vi "Status.vi"(8 "error in (no error)":errorcluster, 11 "Agitator Module State Cluster":T1={"State"=enum."Idle", "Start Time"=timestamp(0 s since 1904-01-01), "Current Time"=timestamp(0 s since 1904-01-01), "Agitator Module Config"={"GUID"="", "Drop Coords"={"Horizontal"=0, "Vertical"=0}, "Process Name"="", "User name"="", "Queue Name"="", "Settings"={"Cycle Period"=500.0, "Agitator Type"="", "Setpoint (µm)"=0.0, "IKA EUROSTAR Settings"={"VISA resource name"="", "Simulated?"=FALSE}}, "Load Count"=0}, "Output Error"=FALSE, "Log Started"=FALSE, "First Iteration"=FALSE, "Data"={"Agitator rpm Value"=0.0}, "Agitator On?"=enum."Off"}) -> (0 "error out":errorcluster, 3 "Agitator Module State Cluster":T1={"State"=enum."Idle", "Start Time"=timestamp(0 s since 1904-01-01), "Current Time"=timestamp(0 s since 1904-01-01), "Agitator Module Config"={"GUID"="", "Drop Coords"={"Horizontal"=0, "Vertical"=0}, "Process Name"="", "User name"="", "Queue Name"="", "Settings"={"Cycle Period"=500.0, "Agitator Type"="", "Setpoint (µm)"=0.0, "IKA EUROSTAR Settings"={"VISA resource name"="", "Simulated?"=FALSE}}, "Load Count"=0}, "Output Error"=FALSE, "Log Started"=FALSE, "First Iteration"=FALSE, "Data"={"Agitator rpm Value"=0.0}, "Agitator On?"=enum."Off"})   [LabVIEW 2018, in "Agitator Module.lvlib" / "Agitator Module Engine.lvlib"]
uses:
  Agitator Module Engine.lvlib
  Feed Module/Controls/Agitator Module State Cluster.ctl
  Pump Module Folder/Measure Instrument/State Enum.ctl
  Feed Module/Controls/Agitator Module Config Cluster.ctl
  <vilib>/Utility/miscctls.llb/LVPoint32TypeDef.ctl
  Feed Module/Controls/Agitator Module Settings Cluster.ctl
  IKA EUROSTAR/IKA EUROSTAR Settings.ctl
  Tag VIs/Tag FGV Operation Enum.ctl
  Shared Variables/Dynamic Shared Variables.lvlib
  Sonic Systems P100/Sonic Systems P100.lvlib
  Pump Module Folder/Measure Instrument/Pump Module Engine.lvlib
  Agitator Module.lvlib
  IKA EUROSTAR/IKA EUROSTAR.lvlib
panel:
  # "Agitator Settings"
  # "Agitator Settings"
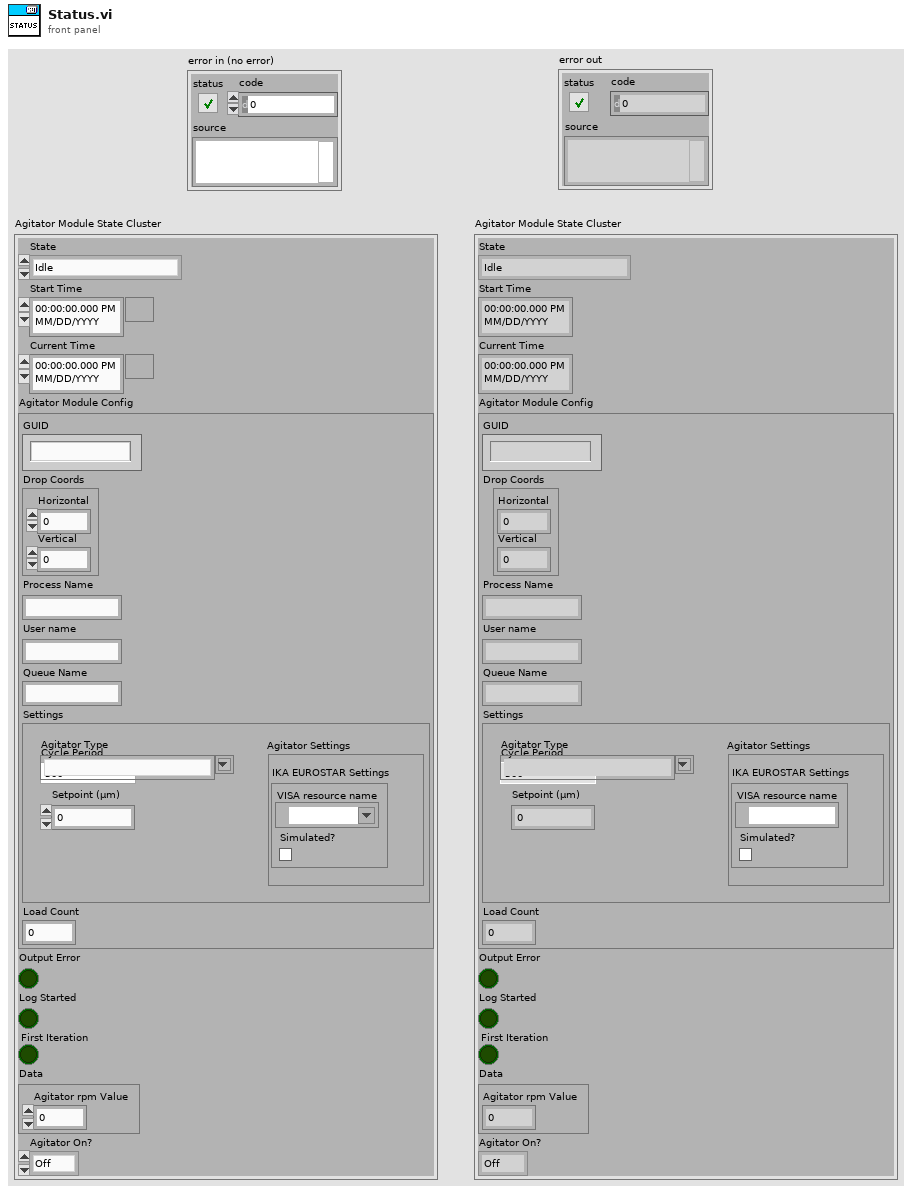
[diagram p1: front panel]
types:
  T1 = typedef "Agitator Module.lvlib/Agitator Module State Cluster.ctl" = cluster{"State":T2, "Start Time":timestamp, "Current Time":timestamp, "Agitator Module Config":T3, "Output Error":bool, "Log Started":bool, "First Iteration":bool, "Data":cluster{"Agitator rpm Value":dbl}, "Agitator On?":enum16{"Off", "On", "Not Initialized", "Over Cutoff"}}
  T2 = typedef "Pump Module.lvlib/Pump Module Engine.lvlib/State Enum.ctl" = enum16{"Measuring", "Idle", "Paused"}
  T3 = typedef "Agitator Module.lvlib/Agitator Module Config Cluster.ctl" = cluster{"GUID":string, "Drop Coords":T4, "Process Name":string, "User name":string, "Queue Name":string, "Settings":T5, "Load Count":i32}
  T4 = typedef "LVPoint32TypeDef.ctl" = cluster{"Horizontal":i32, "Vertical":i32}
  T5 = typedef "Agitator Module.lvlib/Agitator Module Settings Cluster.ctl" = cluster{"Cycle Period":dbl, "Agitator Type":string, "Setpoint (µm)":dbl, "IKA EUROSTAR Settings":T6}
  T6 = typedef "IKA EUROSTAR.lvlib/IKA EUROSTAR Settings.ctl" = cluster{"VISA resource name":refnum<visa-resource-name>, "Simulated?":bool}
  T7 = typedef "Tag FGV Operation Enum.ctl" = enum16{"Init", "Set Notification Queue", "Create Tag", "Commit", "Write Tag (Numeric)", "Write Tag (Boolean)", "Read All Tags", "Read One Tag", "Delete Tag Category", "Set Alarm Parameters (Numeric)", "Set Alarm Parameters (Boolean)", "Enable All Alarms", "Disable All Alarms", "Delete All Tags", "Read Alarms", "Ack Alarm", "Read Alarm Parameters (Numeric)", "Read Alarm Parameters (Boolean)"}
  T8 = cluster{"Amplitude Tag":string, "Power Tag":string, "Output Device Tag":string}
  T9 = typedef "Sonic Systems P100.lvlib/Sonic Systems P100 Settings.ctl" = cluster{"VISA resource name":refnum<visa-resource-name>, "Simulated?":bool}
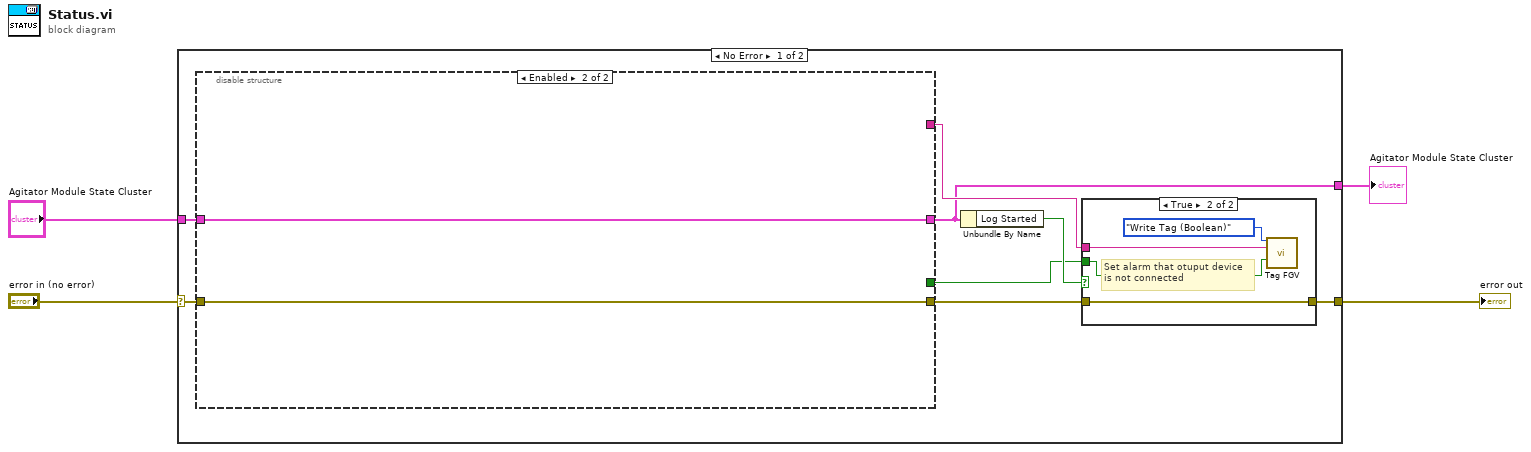
[diagram p0: block diagram]
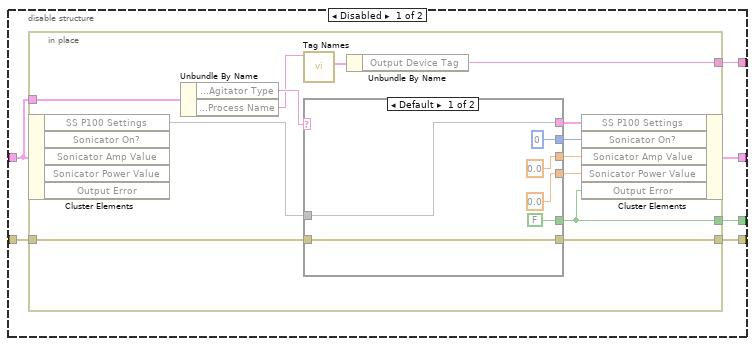
[diagram p2: hidden frame]
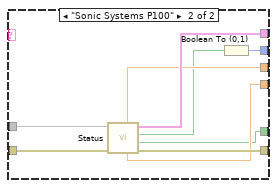
[diagram p3: hidden frame]
diagram:
  n1 = case shown="No Error" "error in (no error)" {
    selector: "error in (no error)" -> [w12 w55]
    tunnel: [w9 w55] -> w3
    tunnel: "Agitator Module State Cluster" -> [w6 w54]
    tunnel: [w5 w54] -> w1
    frame No Error {
      n2 = disable-structure shown="Enabled" {
        disable-tunnel: w12 -> [w18 w47]
        disable-tunnel: [w17 _] -> w11
        disable-tunnel: [w16 w47] -> w10
        disable-tunnel: [w15 _] -> w7
        disable-tunnel: w6 -> [w14 w48]
        disable-tunnel: [w13 w48] -> w5
        frame Disabled {
          n3 = in-place {
            in-place-border: w18 -> [w25]
            in-place-border: [w31] -> w17
            in-place-border: [w26] -> w16
            in-place-border: w14 -> [w21]
            in-place-border: [w22] -> w15
            n4 = in-place-cluster #1(w14) -> ("SS P100 Settings"=w28)  [unwired: 4 out]
            n5 = Unbundle By Name(w21) -> ("Agitator Module Config.Settings.Agitator Type"=w29:string, "Agitator Module Config.Process Name"=w20:string)
            n6 = call "Tag Names.vi"("Process Name"=w20) -> ("SC Tags"=w30:T8)  [unwired: 8 in, 2 out]
            n7 = case shown="Default" w29 {
              tunnel: w28 -> [w37 w46]
              tunnel: [w37 w45] -> w27
              tunnel: [w33 w44] -> w26
              tunnel: w25 -> [w33 w43]
              tunnel: [0.0 ("Amplitude") w42] -> w24
              tunnel: [0.0 ("Power") w41] -> w23
              tunnel: [FALSE ("Connection Error") w40] -> w22
              tunnel: [i16 0 w39] -> w19
              frame Default {
              }
              frame "Sonic Systems P100" {
                n8 = call "Status.vi"("error in (no error)"=w43, "SS P100 Settings In"=w46) -> ("error out"=w44:errorcluster, "Connection Error"=w40:bool, "Running"=w38:bool, "SS P100 Settings Out"=w45:T9, "Power"=w41:dbl, "Amplitude"=w42:dbl)  [unwired: 4 in]
                n9 = Boolean To (0,1)(Boolean=w38) -> (0, 1=w39:i16)
              }
            }
            n10 = Unbundle By Name(w30) -> ("Output Device Tag"=w31:string)
            n11 = in-place-cluster #1("SS P100 Settings"=w27, "Sonicator On?"=w19, "Sonicator Amp Value"=w24, "Sonicator Power Value"=w23, "Output Error"=w22) -> (w13:T1)
          }
        }
        frame Enabled {
        }
      }
      n12 = Unbundle By Name(w5) -> ("Log Started"=w8:bool)
      n13 = case shown="True" w8 {
        tunnel: w11 -> [_ w53]
        tunnel: w10 -> [w49 w52]
        tunnel: [w49 w52] -> w9
        tunnel: w7 -> [_ w50]
        frame False {
        }
        frame True {
          # "Set alarm that otuput device\nis not connected"
          n14 = call "Tag FGV.vi"("Operation"=Tag_FGV_Operation_Enum."Write Tag (Boolean)", "Tag Name"=w53, "Data"=w50) -> ()  [unwired: 5 in, 8 out]
        }
      }
    }
    frame Error {
    }
  }
  "error out" <- w3
  "Agitator Module State Cluster" <- w1
